vi "Get Function Range Output.vi"(8 "error in (no error)":errorcluster, 11 "VISA resource name":refnum<visa-resource-name>) -> (0 "error out":errorcluster, 1 "Autorange enabled":bool, 2 "Output enabled":bool, 3 "VISA resource name out":refnum<visa-resource-name>, 4 "Range {R0-R9}":i32, 5 "Function {F0-F5}":i32, 6 "AC":bool, 7 "DC":bool)   [LabVIEW 2020, in "Datron D4xxx.lvlib"]
doc: "This VI returns selected function, range and output state."
uses:
  Datron D4xxx.lvlib
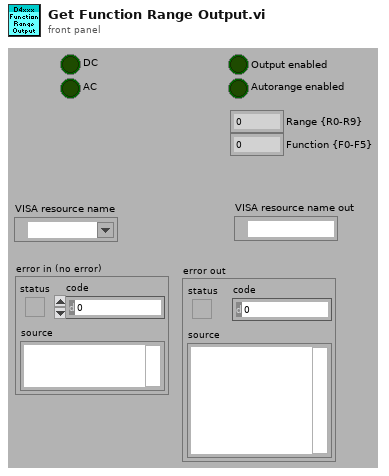
[diagram p1: front panel]
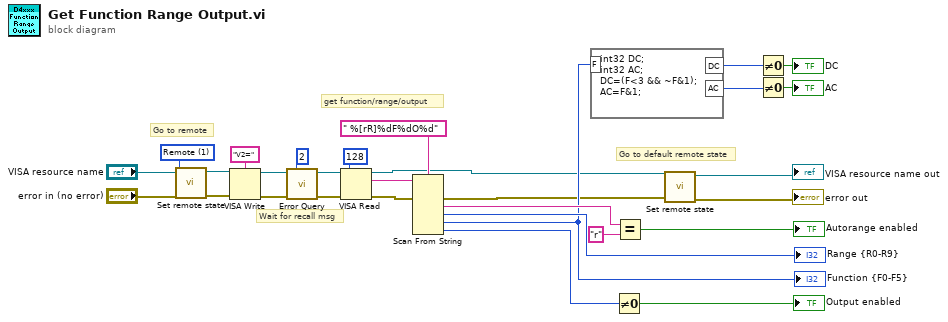
[diagram p0: block diagram]
diagram:
  w10 = u16 1 items=["Local", "Remote", "Default"] ("Remote state")
  # "Wait for recall msg"
  # "Go to default remote state"
  # "Go to remote"
  # "get function/range/output"
  n1 = call "Set remote state.vi"("error in"="error in (no error)", "Remote state"=w10, "VISA resource name"="VISA resource name") -> ("error out"=w14:errorcluster, "VISA resource name out"=w13:refnum<visa-resource-name>)  [unwired: 7 in]
  n2 = VISA Write(VISA resource name=w13, write buffer="V2=", error in (no error)=w14) -> (VISA resource name out=w4:refnum<visa-resource-name>, error out=w5:errorcluster)  [unwired: 1 out]
  n3 = call "Error Query.vi"("error in (no error)"=w5, "Check cycles (11)"=2, "VISA resource name"=w4) -> ("error out"=w7:errorcluster, "VISA resource name out"=w6:refnum<visa-resource-name>)  [unwired: 5 in, 2 out]
  n4 = VISA Read(VISA resource name=w6, byte count=u32 128, error in (no error)=w7) -> (VISA resource name out=w2:refnum<visa-resource-name>, read buffer=w26:string, error out=w28:errorcluster)  [unwired: 1 out]
  n5 = Scan From String(format string=" %[rR]%dF%dO%d", input string=w26, error in=w28) -> (error out=w1:errorcluster, output 1=w25:string, output 2=→"Range {R0-R9}":i32, output 3=w19:i32, output 4=w21:i32)  [unwired: 5 in, 2 out]
  "Function {F0-F5}" <- w19
  n6 = formula code="int32 DC;\nint32 AC;\nDC=(F<3 && ~F&1);\nAC=F&1;"("F"=w19) -> ("DC"=w17:i32, "AC"=w15:i32)
  n7 = Not Equal To 0?(x=w21) -> (x != 0?=→"Output enabled":bool)
  n8 = Equal?(x=w25, y="r") -> (x = y?=→"Autorange enabled":bool)
  n9 = call "Set remote state.vi"("error in"=w1, "VISA resource name"=w2) -> ("error out"=→"error out":errorcluster, "VISA resource name out"=→"VISA resource name out":refnum<visa-resource-name>)  [unwired: 8 in]
  n10 = Not Equal To 0?(x=w17) -> (x != 0?=→"DC":bool)
  n11 = Not Equal To 0?(x=w15) -> (x != 0?=→"AC":bool)
